vi "Init.vi"(8 "error in (no error)":errorcluster, 10 "Params":variant, 11 "NI PXI Trigger in":refnum<class "NI PXI Trigger.lvclass">) -> (0 "error out":errorcluster, 3 "NI PXI Trigger out":refnum<class "NI PXI Trigger.lvclass">)   [LabVIEW 2020, in "NI DAQmx.lvlib" / "NI PXI Trigger.lvclass"]
uses:
  NI PXI Trigger.lvclass
  PXI Trigger config.ctl
  NI PXI Trigger.lvclass/NI PXI Trigger.ctl
  <vilib>/DAQmx/create/channels.llb/DAQmx Create Channel (CO-Pulse Generation-Frequency).vi
  <vilib>/DAQmx/configure/timing.llb/DAQmx Timing (Implicit).vi
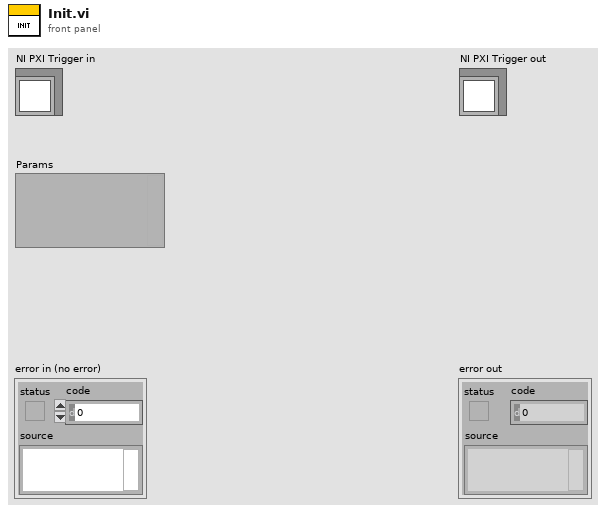
[diagram p1: front panel]
types:
  T1 = typedef "PXI Trigger config.ctl" = cluster{"counter output":string, "source terminal":string, "destination terminal":string}
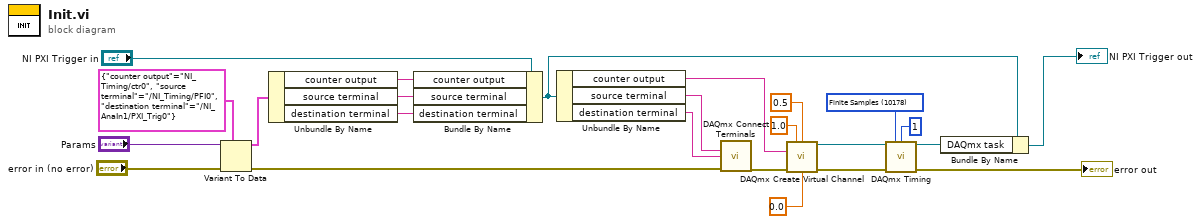
[diagram p0: block diagram]
diagram:
  w20 = 10178 items=["Finite Samples"=10178, "Continuous Samples"=10123, "Hardware Timed Single Point"=12522] ("sample mode")
  n1 = Variant To Data(error in="error in (no error)", type=T1 {"counter output"="NI_Timing/ctr0", "source terminal"="/NI_Timing/PFI0", "destination terminal"="/NI_AnaIn1/PXI_Trig0"} ("Cluster of class private data"), Variant="Params") -> (data=w10:T1, error out=w14:errorcluster)
  n2 = Unbundle By Name(w10) -> ("counter output"=w9:string, "source terminal"=w8:string, "destination terminal"=w7:string)
  n3 = Bundle By Name(cluster="NI PXI Trigger in", "counter output"=w9, "source terminal"=w8, "destination terminal"=w7) -> (w3:refnum<class "NI PXI Trigger.lvclass">)
  n4 = Unbundle By Name(w3) -> ("counter output"=w4:tag, "source terminal"=w6:tag, "destination terminal"=w5:tag)
  n5 = call <vilib>:"DAQmx Connect Terminals.vi"("source terminal"=w6, "destination terminal"=w5, "error in"=w14) -> ("error out"=w16:errorcluster)  [unwired: 12 in]
  n6 = call-poly <vilib>:"DAQmx Create Virtual Channel.vi"("frequency"=1.0, "duty cycle"=0.5, "counter"=w4, "error in"=w16, "initial delay"=0.0) -> ("task out"=w18:refnum<k21>, "error out"=w19:errorcluster)  [unwired: 9 in]
  n7 = call-poly <vilib>:"DAQmx Timing.vi"("task/channels in"=w18, "sample mode"=w20, "samples per channel"=1, "error in"=w19) -> ("task out"=w1:refnum<k21>, "error out"=→"error out":errorcluster)  [unwired: 10 in]
  n8 = Bundle By Name(cluster=w3, "DAQmx task"=w1) -> (→"NI PXI Trigger out":refnum<class "NI PXI Trigger.lvclass">)
